vi "GetAllBufferedGRIMMData.vi"(0 "NumberOfDataPoints":i32, 1 "Duration":i32, 2 "Format":string caption="Format (use accept header)", 4 "LabVIEW Web Service Request":refnum<class "Web Request.lvclass">) -> ()   [LabVIEW 2013]
uses:
  <vilib>/wsapi/Web Request.lvclass
  GRIMM/GRIMMmeasurementEnum.ctl
  GRIMM/GRIMMCurrentCountsPerBin.ctl
panel:
  # "Use the Web Service Request input terminal to call the VIs on the Web Services palette. Do not remove it from the connector pane unless you don't need access to the palette."
  # "Each additional control wired to the connector pane will be available as an input in the URL. To include an indicator in terminal-mode output (the default setting), it must also be wired to the connector pane."
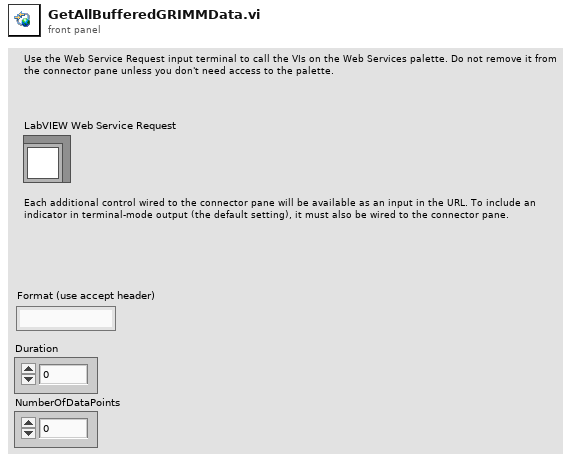
[diagram p1: front panel]
types:
  T1 = typedef "GRIMMCurrentCountsPerBin.ctl" = cluster{"dateTime":string, "CountsPerBin":dbl[]}
  T2 = cluster{"Duration(counts)":i32, "NumberOfDataPoints":i32}
  T3 = typedef "GRIMMmeasurementEnum.ctl" = enum16{"GetBufferedData", "Get CurrentNvsBin WebService", "Save Raw to file", "Get NvsDiameter", "Get DNDlogDPVsDiameter", "Get CountsVsTime", "Get Raw Data", "InsertMeasurement", "Init"}
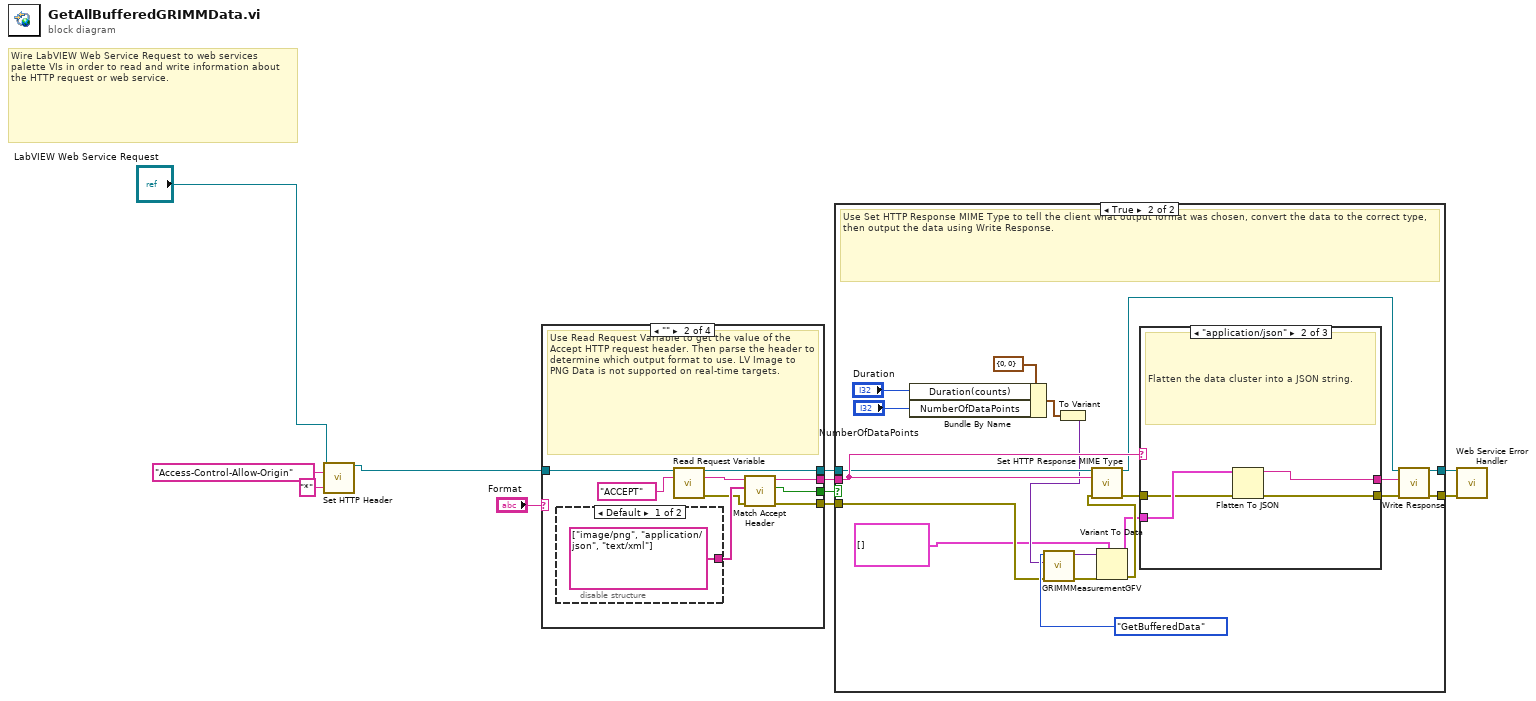
[diagram p0: block diagram]
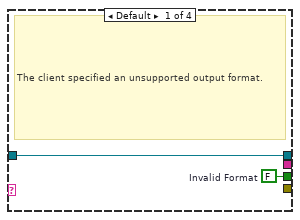
[diagram p2: hidden frame]
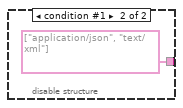
[diagram p3: hidden frame]
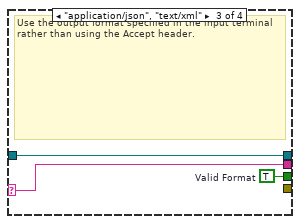
[diagram p4: hidden frame]
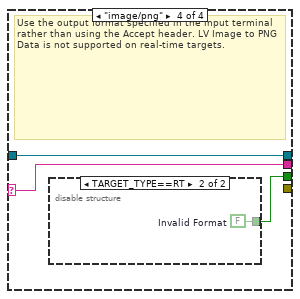
[diagram p5: hidden frame]
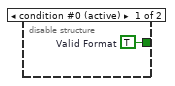
[diagram p6: hidden frame]
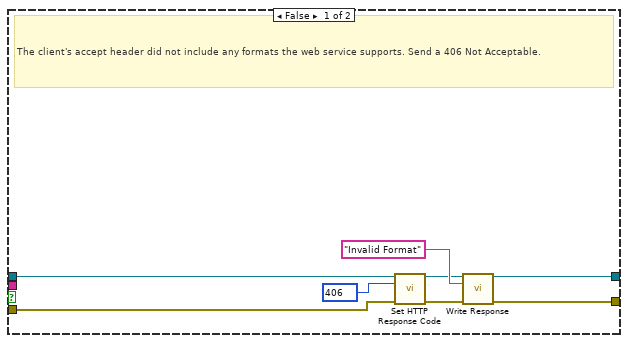
[diagram p7: hidden frame]
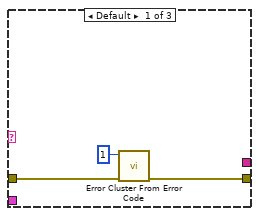
[diagram p8: hidden frame]
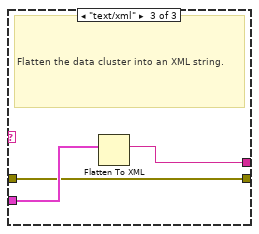
[diagram p9: hidden frame]
diagram:
  # "Wire LabVIEW Web Service Request to web services palette VIs in order to read and write information about the HTTP request or web service."
  n1 = call <vilib>:"Set HTTP Header.vi"("LabVIEW Web Service Request"="LabVIEW Web Service Request", "header"="Access-Control-Allow-Origin", "header value"="*") -> ("LabVIEW Web Service Request out"=w4:refnum<class "Web Request.lvclass">)  [unwired: 11 in, 1 out]
  n2 = case shown="\"\"" "Format" {
    selector: "Format" -> [_ _ w26 w29]
    tunnel: w4 -> [w13 w14 w27 w30]
    tunnel: [w12 w19 w25 w28] -> w11
    tunnel: [w13 w18 w27 w30] -> w10
    tunnel: [_ w16 _ _] -> w9
    tunnel: [_ w15 w26 w29] -> w8
    frame Default {
      w12 = FALSE  # Invalid Format
      # "The client specified an unsupported output format."
    }
    frame "" {
      # "Use Read Request Variable to get the value of the Accept HTTP request header. Then parse the header to determine which output format to use. LV Image to PNG Data is not supported on real-time targets."
      n3 = disable-structure shown="Default" {
        disable-tunnel: [string[] ["image/png", "application/json", "text/xml"] ("Valid Media Types") string[] ["application/json", "text/xml"] ("Valid Media Types")] -> w20
        frame condition #0 (active) {
        }
        frame condition #1 {
        }
      }
      n4 = call <vilib>:"Read Request Variable.vi"("LabVIEW Web Service Request"=w14, "variable name"="ACCEPT") -> ("LabVIEW Web Service Request out"=w18:refnum<class "Web Request.lvclass">, "value"=w21:string, "error out"=w17:errorcluster)  [unwired: 11 in]
      n5 = call "Match Accept Header.vi"("error in (no error)"=w17, "Valid Media Types"=w20, "Accept Value"=w21) -> ("error out"=w16:errorcluster, "Matched?"=w19:bool, "Matched Media Type"=w15:string)  [unwired: 6 in]
    }
    frame "application/json", "text/xml" {
      w25 = TRUE  # Valid Format
      # "Use the output format specified in the input terminal rather than using the Accept header."
    }
    frame "image/png" {
      # "Use the output format specified in the input terminal rather than using the Accept header. LV Image to PNG Data is not supported on real-time targets."
      n6 = disable-structure shown="TARGET_TYPE==RT" {
        disable-tunnel: [w31 w32] -> w28
        frame condition #0 (active) {
          w31 = TRUE  # Valid Format
        }
        frame condition #1 {
          w32 = FALSE  # Invalid Format
        }
      }
    }
  }
  n7 = case shown="True" w11 {
    tunnel: w10 -> [w34 w54]
    tunnel: w9 -> [w39 w47]
    tunnel: w8 -> [_ w59]
    tunnel: [w36 w56] -> w7
    tunnel: [w35 w55] -> w6
    frame False {
      w40 = 406 items=["100"=100, "101"=101, "200"=200, "201"=201, "202"=202, "203"=203, "204"=204, "205"=205, "206"=206, "300"=300, "301"=301, "302"=302, "303"=303, "304"=304, "305"=305, "306"=306, "307"=307, "400"=400, "401"=401, "402"=402, "403"=403, "404"=404, "405"=405, "406"=406, "407"=407, "408"=408, "409"=409, "410"=410, "411"=411, "412"=412, "413"=413, "414"=414, "415"=415, "416"=416, "417"=417, "500"=500, "501"=501, "502"=502, "503"=503, "504"=504, "505"=505] ("response code (200)")
      # "The client's accept header did not include any formats the web service supports. Send a 406 Not Acceptable."
      n8 = call <vilib>:"Set HTTP Response Code.vi"("LabVIEW Web Service Request"=w34, "response code (200)"=w40, "error in (no error)"=w39) -> ("LabVIEW Web Service Request out"=w33:refnum<class "Web Request.lvclass">, "error out"=w38:errorcluster)  [unwired: 11 in]
      n9 = call <vilib>:"Write Response.vi"("LabVIEW Web Service Request"=w33, "response string"="Invalid Format", "error in (no error)"=w38) -> ("LabVIEW Web Service Request out"=w35:refnum<class "Web Request.lvclass">, "error out"=w36:errorcluster)  [unwired: 11 in]
    }
    frame True {
      # "Use Set HTTP Response MIME Type to tell the client what output format was chosen, convert the data to the correct type, then output the data using Write Response."
      n10 = Bundle By Name(cluster=T2 {"Duration(counts)"=0, "NumberOfDataPoints"=0}, "Duration(counts)"="Duration", "NumberOfDataPoints"="NumberOfDataPoints") -> (w45:T2)
      n11 = To Variant(anything=w45) -> (Variant=w44:variant)
      n12 = call "GRIMMMeasurementGFV.vi"("error in (no error)"=w47, "Variant in"=w44, "GRIMMMeasEnum"=GRIMMmeasurementEnum."GetBufferedData") -> ("error out"=w48:errorcluster, "Variant out"=w49:variant)  [unwired: 7 in]
      n13 = Variant To Data(error in=w48, type=T1[] [], Variant=w49) -> (data=w51:T1[], error out=w52:errorcluster)
      n14 = call <vilib>:"Set HTTP Response MIME Type.vi"("LabVIEW Web Service Request"=w54, "MIME type (text/html)"=w59, "error in (no error)"=w52) -> ("LabVIEW Web Service Request out"=w53:refnum<class "Web Request.lvclass">, "error out"=w60:errorcluster)  [unwired: 11 in]
      n15 = case shown="\"application/json\"" w59 {
        tunnel: w60 -> [w63 w66 w69]
        tunnel: w51 -> [_ w67 w70]
        tunnel: [w62 w64 w69] -> w57
        tunnel: [_ w65 w68] -> w58
        frame Default {
          n16 = call <vilib>:"Error Cluster From Error Code.vi"("error in (no error)"=w63, "error code (0)"=1) -> ("error out"=w62:errorcluster)  [unwired: 7 in]
        }
        frame "application/json" {
          # "Flatten the data cluster into a JSON string."
          n17 = Flatten To JSON(anything=w67, error in (no error)=w66) -> (JSON string=w65:string, 11:w64:errorcluster)  [unwired: 1 in]
        }
        frame "text/xml" {
          # "Flatten the data cluster into an XML string."
          n18 = Flatten To XML(anything=w70) -> (xml string=w68:string)
        }
      }
      n19 = call <vilib>:"Write Response.vi"("LabVIEW Web Service Request"=w53, "response string"=w58, "error in (no error)"=w57) -> ("LabVIEW Web Service Request out"=w55:refnum<class "Web Request.lvclass">, "error out"=w56:errorcluster)  [unwired: 11 in]
    }
  }
  n20 = call "Web Service Error Handler.vi"("LabVIEW Web Service Request"=w6, "error in (no error)"=w7) -> ()  [unwired: 12 in, 2 out]
